vi "Read Desired Temperature.vi"(11 "冷却器的控制器输入":refnum<class "Cooler Controller.lvclass">) -> (2 "待维持的温度":dbl=75.0)   [LabVIEW 2015, in "Cooler Controller.lvlib" / "Cooler Controller.lvclass"]
uses:
  Cooler Controller.lvclass
  Cooler Controller.lvclass/Cooler Controller.ctl
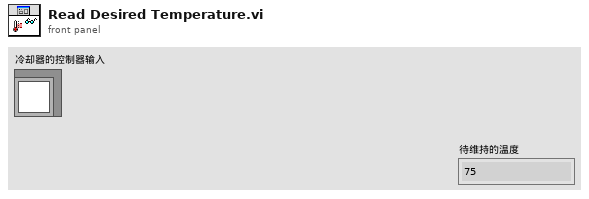
[diagram p1: front panel]
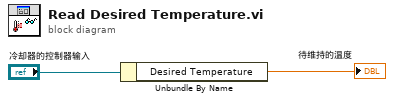
[diagram p0: block diagram]
diagram:
  n1 = Unbundle By Name("冷却器的控制器输入") -> ("Desired Temperature"=→"待维持的温度":dbl)
